vi "single sweep - rus clean up.vi"(6 "Zero amplitude at the end":bool=TRUE, 7 "Stop user event":refnum<user-event>, 8 "error in (no error)":errorcluster, 11 "RUS settings":T1={"NI-DAQ lockin settings"={"Samples per sine wave"=0, "Sine waves per freq step"=0, "Output Representation"=enum."Real/Imaginary", "Low-pass filter"=enum."Butterworth", "Ranges and couplings "=[]}, "Fast swep settings"={"Update rate (Hz)"=250.0, "Start F, Hz"=200000.0, "Stop F"=1700000.0, "Number of points"=30000, "Amplitude"=2.1, "Init&amplitude"=TRUE, "IF"=1000.0, "Time constant"=0.1}, "Pre-sweep delay, s"=0.0, "Lockin mode"=enum."NI-DAQ", "SR Lockin"="GPIB0::10::INSTR", "DAQmx Device"="Dev3", "Clock Multiplier"=64, "Fast Sweep Data Out"={"DO clock task"="", "DO task"="", "Update clock task"="", "DAQ lockin task"="", "Pre-sweep counter task"=""}, "Lockin Range, V"=0.0, "F Array"=[], "Freq. update clock terminal"="", "DO Clock Rate (Hz)"=5000000.0, "ADC clock terminal"="/PFI4", "Pre-sweep counter terminal"="", "Samples per read"=10, "DO clock terminal"="", "Pre-sweep points"=0, "F points per write"=1000, "Total sweep time, s"=0.0, "Initial SYNTH phase"=0.0, "Record IF"=FALSE, "Save data settings"={"Save data"=TRUE, "Data Root Path"=path "", "File Prefix"="", "File Format"=enum."ASCII", "Save column names"=TRUE, "File Comments"="<Description of the current file>", "User/Prj"="<User Name/Project Description>"}, "Data file path"=path "", "New data user event"=refnum, "Stop user event"=refnum, "Number of channels"=1, "Auto-phase"=FALSE, "RP Transeiver"=refnum} {"Lockin Range, V" format="%#_6e"; "Fast swep settings"."IF" format="%#_6p"; "Fast swep settings"."Amplitude" min=0.0 max=2.5; "Fast swep settings"."Number of points" format="%.0p"; "Fast swep settings"."Stop F" format="%#_6p"; "Fast swep settings"."Start F, Hz" format="%#_6p"; "Fast swep settings"."Update rate (Hz)" format="%0.2f"; "NI-DAQ lockin settings"."Ranges and couplings"."Coupling" items=["default"=-1, "RSE"=10083, "NRSE"=10078, "Differential"=10106, "Pseudodifferential"=12529]}) -> (0 "error out":errorcluster, 1 "STD status byte":u8 format="%08b", 2 "Error status byte\n(bit 5 - FAST aborted)":u8 format="%08b", 3 "RUS settings out":T1={"NI-DAQ lockin settings"={"Samples per sine wave"=0, "Sine waves per freq step"=0, "Output Representation"=enum."Real/Imaginary", "Low-pass filter"=enum."Butterworth", "Ranges and couplings "=[]}, "Fast swep settings"={"Update rate (Hz)"=250.0, "Start F, Hz"=200000.0, "Stop F"=1700000.0, "Number of points"=30000, "Amplitude"=2.1, "Init&amplitude"=TRUE, "IF"=1000.0, "Time constant"=0.1}, "Pre-sweep delay, s"=0.0, "Lockin mode"=enum."NI-DAQ", "SR Lockin"="GPIB0::10::INSTR", "DAQmx Device"="Dev3", "Clock Multiplier"=64, "Fast Sweep Data Out"={"DO clock task"="", "DO task"="", "Update clock task"="", "DAQ lockin task"="", "Pre-sweep counter task"=""}, "Lockin Range, V"=0.0, "F Array"=[], "Freq. update clock terminal"="", "DO Clock Rate (Hz)"=5000000.0, "ADC clock terminal"="/PFI4", "Pre-sweep counter terminal"="", "Samples per read"=10, "DO clock terminal"="", "Pre-sweep points"=0, "F points per write"=1000, "Total sweep time, s"=0.0, "Initial SYNTH phase"=0.0, "Record IF"=FALSE, "Save data settings"={"Save data"=TRUE, "Data Root Path"=path "", "File Prefix"="", "File Format"=enum."ASCII", "Save column names"=TRUE, "File Comments"="<Description of the current file>", "User/Prj"="<User Name/Project Description>"}, "Data file path"=path "", "New data user event"=refnum, "Stop user event"=refnum, "Number of channels"=1, "Auto-phase"=FALSE, "RP Transeiver"=refnum} {"Lockin Range, V" format="%#_6e"; "Fast swep settings"."IF" format="%#_6p"; "Fast swep settings"."Amplitude" min=0.0 max=2.5; "Fast swep settings"."Number of points" format="%.0p"; "Fast swep settings"."Stop F" format="%#_6p"; "Fast swep settings"."Start F, Hz" format="%#_6p"; "Fast swep settings"."Update rate (Hz)" format="%0.2f"; "NI-DAQ lockin settings"."Ranges and couplings"."Coupling" items=["default"=-1, "RSE"=10083, "NRSE"=10078, "Differential"=10106, "Pseudodifferential"=12529]})   [LabVIEW 2016]
uses:
  resonant_ultrasound/Libraries/RUS/Controls/RUS NI-DAQ Lockin Settings.ctl
  resonant_ultrasound/Libraries/RUS/Controls/Sweep settings.ctl
  resonant_ultrasound/Libraries/RUS/Controls/RUS settings.ctl
  NHMFL_Core/Libraries/File/Controls/File formats.ctl
  NHMFL_Core/Libraries/File/Controls/Save data settings.ctl
  resonant_ultrasound/Libraries/RUS/Controls/Lockin mode.ctl
  NHMFL_Core/Libraries/Red Pitaya/RP Core/RP Transceiver/RP Transceiver.lvclass
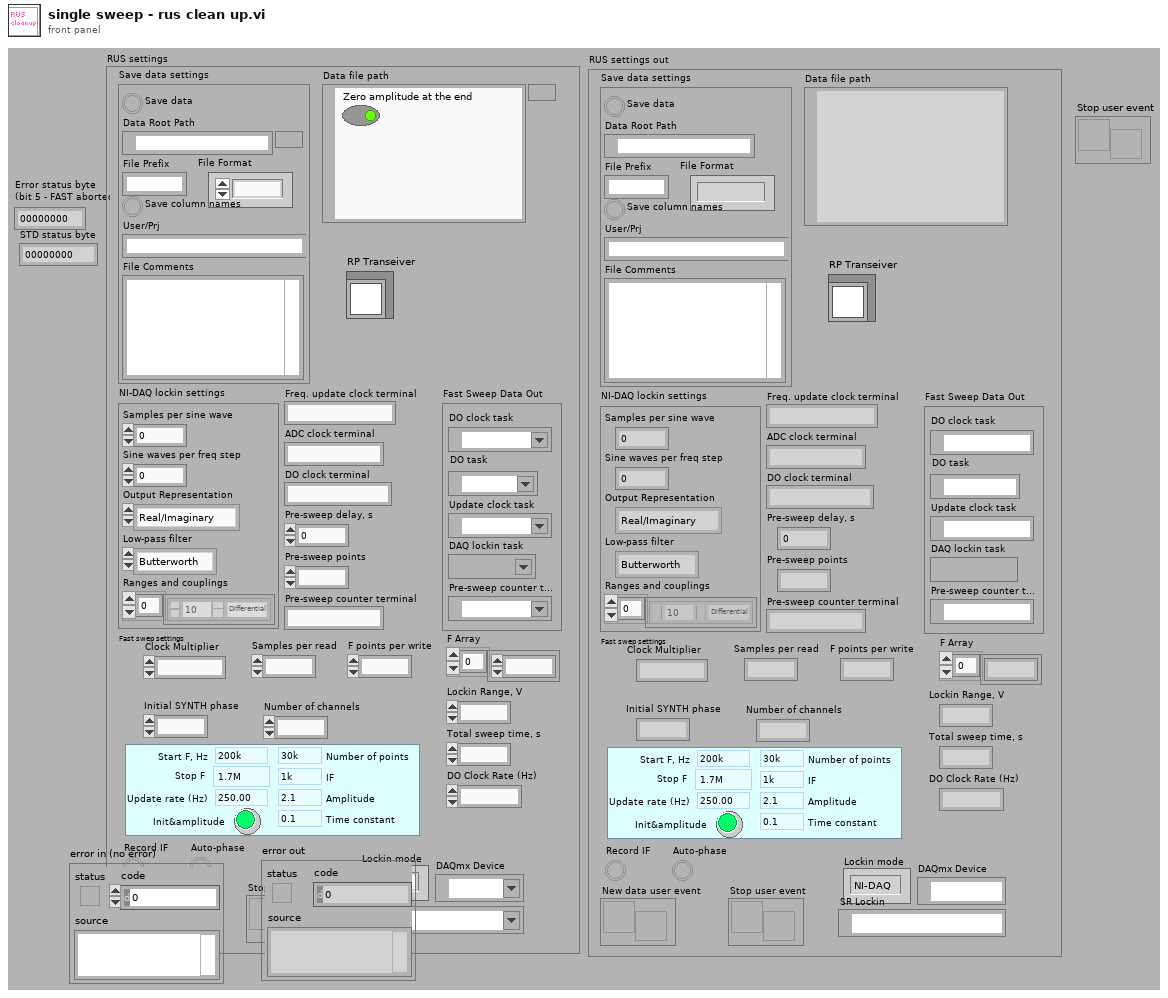
[diagram p1: front panel]
types:
  T1 = typedef "RUS settings.ctl" = cluster{"NI-DAQ lockin settings":T2, "Fast swep settings":T3, "Pre-sweep delay, s":dbl, "Lockin mode":T4, "SR Lockin":refnum<visa-resource-name>, "DAQmx Device":tag, "Clock Multiplier":i32, "Fast Sweep Data Out":cluster{"DO clock task":refnum<k21>, "DO task":refnum<k21>, "Update clock task":refnum<k21>, "DAQ lockin task":refnum<k21>, "Pre-sweep counter task":refnum<k21>}, "Lockin Range, V":sgl, "F Array":dbl[], "Freq. update clock terminal":string, "DO Clock Rate (Hz)":dbl, "ADC clock terminal":string, "Pre-sweep counter terminal":string, "Samples per read":i32, "DO clock terminal":string, "Pre-sweep points":i32, "F points per write":i32, "Total sweep time, s":dbl, "Initial SYNTH phase":dbl, "Record IF":bool, "Save data settings":T5, "Data file path":path, "New data user event":refnum<user-event>, "Stop user event":refnum<user-event>, "Number of channels":i32, "Auto-phase":bool, "RP Transeiver":refnum<class "RP Transceiver.lvclass">}
  T2 = typedef "RUS NI-DAQ Lockin Settings.ctl" = cluster{"Samples per sine wave":i32, "Sine waves per freq step":i32, "Output Representation":enum16{"Real/Imaginary", "Polar"}, "Low-pass filter":enum16{"No filtering", "Butterworth", "Bessel"}, "Ranges and couplings ":cluster{"Range":dbl, "Coupling":i32}[]}
  T3 = typedef "Sweep settings.ctl" = cluster{"Update rate (Hz)":dbl, "Start F, Hz":dbl, "Stop F":dbl, "Number of points":i32, "Amplitude":dbl, "Init&amplitude":bool, "IF":dbl, "Time constant":dbl}
  T4 = typedef "Lockin mode.ctl" = enum16{"SRS", "NI-DAQ", "Pitaya"}
  T5 = typedef "Save data settings.ctl" = cluster{"Save data":bool, "Data Root Path":path, "File Prefix":string, "File Format":T6, "Save column names":bool, "File Comments":string, "User/Prj":string}
  T6 = typedef "File formats.ctl" = enum16{"TDMS", "ASCII", "BINARY"}
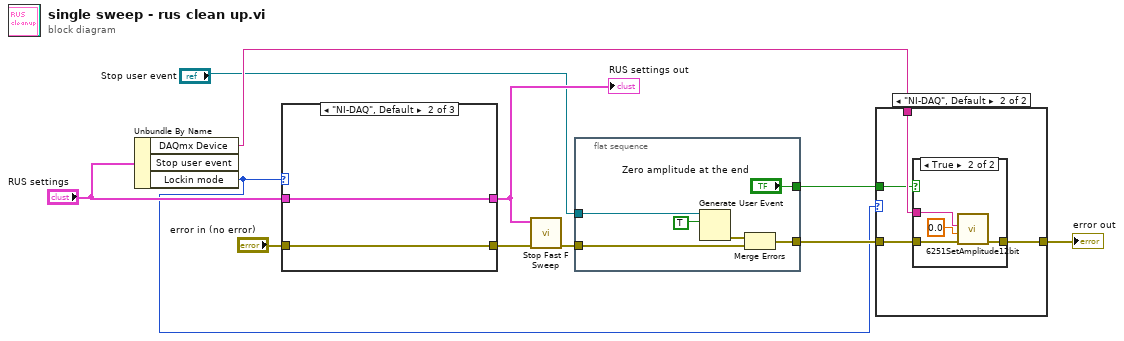
[diagram p0: block diagram]
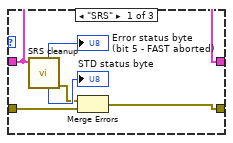
[diagram p4: hidden frame]
diagram:
  n1 = Unbundle By Name("RUS settings") -> ("DAQmx Device"=w6:tag, "Lockin mode"=w1:T4)  [unwired: 1 out]
  n2 = case shown="\"NI-DAQ\", Default" w1 {
    tunnel: "RUS settings" -> [w14 w19 w21]
    tunnel: [w13 w18 w20] -> w9
    tunnel: [w14 w19 w21] -> w3
    tunnel: "error in (no error)" -> [w12 w18 w20]
    frame "SRS" {
      n3 = call "SRS cleanup.vi"("RUS settings"=w14) -> ("error out"=w15:errorcluster, "STD status byte"=→"STD status byte":u8, "Error status byte\n(bit 5 - FAST aborted)"=→"Error status byte\n(bit 5 - FAST aborted)":u8)  [unwired: 7 in, 1 out]
      n4 = Merge Errors(w15, w12) -> (w13:errorcluster)
    }
    frame "NI-DAQ", Default {
    }
    frame "Pitaya" {
    }
  }
  "RUS settings out" <- w3
  n5 = call "Stop Fast F Sweep.vi"("error in (no error)"=w9, "RUS settings"=w3) -> ("error out"=w8:errorcluster)  [unwired: 1 in, 8 out]
  n6 = flat-sequence {
    tunnel: [w26] -> w7
    tunnel: "Stop user event" -> [w27]
    tunnel: w8 -> [w23]
    tunnel: ["Zero amplitude at the end"] -> w5
    frame #0 {
      n7 = Generate User Event(user event=w27, event data cluster=TRUE ("element")) -> (error out=w22:errorcluster)  [unwired: 2 in, 1 out]
      n8 = Merge Errors(w22, w23) -> (w26:errorcluster)
    }
  }
  n9 = case shown="\"NI-DAQ\", Default" w1 {
    tunnel: w7 -> [w28 w32]
    tunnel: w6 -> [_ w31]
    tunnel: w5 -> [_ w30]
    tunnel: [w28 w29] -> w4
    frame "Pitaya" {
    }
    frame "NI-DAQ", Default {
      n10 = case shown="True" w30 {
        tunnel: w32 -> [w33 w37]
        tunnel: [w33 w36] -> w29
        tunnel: w31 -> [_ w35]
        frame False {
        }
        frame True {
          n11 = call "6251SetAmplitude12bit.vi"("error in (no error)"=w37, "0 to 2.1 VRMS"=0.0, "DAQmx Device Name"=w35) -> ("error out"=w36:errorcluster)  [unwired: 8 out]
        }
      }
    }
  }
  "error out" <- w4
